vi "BMU诊断标定.vi"(8 "CAN端口":u16(ring), 9 "设备索引号":u16(ring), 10 "CAN卡类型":u32(ring)=21) -> ()   [LabVIEW 2013] (continued)
                n2409 = local write "正级继电器 9"(w2970) -> ()
                n2410 = local write "主从选择"(enum32{"主板", "从板"}."主板" ("主从选择")) -> ()
              }
              frame #1 {
                n2411 = case shown="真" w2980 {
                  selector: w2980 -> [w2995 w3015]
                  tunnel: [w2994 w3014] -> w2979
                  tunnel: [w2982 w3002] -> w2974
                  frame False {
                    w2990 = 256.0 ("y")
                    w2982 = u32 2 ("命令序号")
                    w2994 = u8 192 ("命令")
                    n2412 = local read "动作保持时间"() -> (w2991:dbl)
                    n2413 = Quotient & Remainder(x=w2991, y=w2990) -> (x-y*floor(x/y)=w2983:dbl, floor(x/y)=w2987:dbl)
                    n2414 = Quotient & Remainder(x=w2987, y=w2990) -> (x-y*floor(x/y)=w2984:dbl, floor(x/y)=w2988:dbl)
                    n2415 = Quotient & Remainder(x=w2988, y=w2990) -> (x-y*floor(x/y)=w2985:dbl, floor(x/y)=w2989:dbl)
                    n2416 = local read "设备索引号"() -> (w2999:u16)
                    n2417 = local read "CAN卡类型"() -> (w3000:u32)
                    n2418 = local read "CAN端口"() -> (w2998:u16)
                    n2419 = Boolean To (0,1)(Boolean=w2995) -> (0, 1=w2992:i16)
                    n2420 = Quotient & Remainder(x=w2989, y=w2990) -> (x-y*floor(x/y)=w2986:dbl)  [unwired: 1 out]
                    n2421 = Build Array(i16 1 ("元素"), w2992, w2986, w2985, w2984, w2983, 0.0 ("元素")) -> (w2996:dbl[])
                    n2422 = call "多帧发送机制(EV05).vi"("can卡类型"=w3000, "设备索引号"=w2999, "CAN端口"=w2998, "命令"=w2994, "板号"=u8 0, "命令序号"=w2982, "输入数据"=w2996) -> ()  [unwired: 1 in, 12 out]
                  }
                  frame True {
                    w3010 = 256.0 ("y")
                    w3002 = u32 2 ("命令序号")
                    w3014 = u8 192 ("命令")
                    n2423 = local read "动作保持时间"() -> (w3011:dbl)
                    n2424 = Quotient & Remainder(x=w3011, y=w3010) -> (x-y*floor(x/y)=w3003:dbl, floor(x/y)=w3007:dbl)
                    n2425 = Quotient & Remainder(x=w3007, y=w3010) -> (x-y*floor(x/y)=w3004:dbl, floor(x/y)=w3008:dbl)
                    n2426 = Quotient & Remainder(x=w3008, y=w3010) -> (x-y*floor(x/y)=w3005:dbl, floor(x/y)=w3009:dbl)
                    n2427 = local read "设备索引号"() -> (w3019:u16)
                    n2428 = local read "CAN卡类型"() -> (w3020:u32)
                    n2429 = local read "CAN端口"() -> (w3018:u16)
                    n2430 = Boolean To (0,1)(Boolean=w3015) -> (0, 1=w3012:i16)
                    n2431 = Quotient & Remainder(x=w3009, y=w3010) -> (x-y*floor(x/y)=w3006:dbl)  [unwired: 1 out]
                    n2432 = Build Array(i16 1 ("元素"), w3012, w3006, w3005, w3004, w3003, 0.0 ("元素")) -> (w3016:dbl[])
                    n2433 = call "多帧发送机制(EV05).vi"("can卡类型"=w3020, "设备索引号"=w3019, "CAN端口"=w3018, "命令"=w3014, "板号"=u8 0, "命令序号"=w3002, "输入数据"=w3016) -> ()  [unwired: 1 in, 12 out]
                  }
                }
                n2434 = local write "命令序号"(w2974) -> ()
                n2435 = local write "命令"(w2979) -> ()
                n2436 = local write "控制1"(TRUE ("控制1")) -> ()
                n2437 = local write "写?"(FALSE ("写?")) -> ()
                n2438 = local write "消除"(TRUE ("消除")) -> ()
                n2439 = global write "EV05全局变量1.vi" "流控帧 2"(TRUE ("流控帧 2")) -> ()
                n2440 = global write "EV05全局变量1.vi" "流控帧"(FALSE ("流控帧")) -> ()
              }
              frame #2 {
                n2441 = flat-sequence {
                  tunnel: [w3022] -> w3021
                  tunnel: w3021 -> [w3029]
                  frame #0 {
                    n2442 = while {
                      tunnel: [w3023] -> w3022
                      i -> [w3027]
                      stop <- w3024 stop-if-true
                      n2443 = local read "继电器超时处理"() -> (w3023:bool)
                      n2444 = Greater Or Equal?(x=w3027, y=20) -> (x >= y?=w3025:bool)
                      n2445 = Wait Until Next ms Multiple(millisecond multiple=u32 100 ("毫秒倍数")) -> ()  [unwired: 1 out]
                      n2446 = Or(x=w3023, y=w3025) -> (x .or. y?=w3024:bool)
                    }
                  }
                  frame #1 {
                    n2447 = case shown="假" w3029 {
                      frame False {
                        n2448 = local read "DO1"() -> (w3031:bool)
                        n2449 = Not(x=w3031) -> (.not. x?=w3030:bool)
                        n2450 = local write "DO1"(w3030) -> ()
                        n2451 = One Button Dialog(message="DO控制处理超时" ("消息"), button name ("OK")="是" ("按钮名称（“确定”）")) -> ()  [unwired: 1 out]
                      }
                      frame True {
                      }
                    }
                  }
                }
              }
            }
          }
          event "DO2": Value Change {
            n2452 = event-data() -> ("NewVal"=w3034:bool)  [unwired: 6 out]
            n2453 = stacked-sequence {
              tunnel: w3034 -> [_ w3047 _]
              frame #0 {
                w3037 = FALSE ("清BUFF")
                n2454 = local write "继电器超时处理"(FALSE ("继电器超时处理")) -> ()
                n2455 = local write "主从选择"(enum32{"主板", "从板"}."主板" ("主从选择")) -> ()
                n2456 = local write "清BUFF"(w3037) -> ()
                n2457 = local write "正级继电器 10"(w3037) -> ()
              }
              frame #1 {
                n2458 = case shown="真" w3047 {
                  selector: w3047 -> [w3062 w3082]
                  tunnel: [w3061 w3081] -> w3046
                  tunnel: [w3049 w3069] -> w3041
                  frame False {
                    w3057 = 256.0 ("y")
                    w3049 = u32 2 ("命令序号")
                    w3061 = u8 192 ("命令")
                    n2459 = local read "动作保持时间"() -> (w3058:dbl)
                    n2460 = Quotient & Remainder(x=w3058, y=w3057) -> (x-y*floor(x/y)=w3050:dbl, floor(x/y)=w3054:dbl)
                    n2461 = Quotient & Remainder(x=w3054, y=w3057) -> (x-y*floor(x/y)=w3051:dbl, floor(x/y)=w3055:dbl)
                    n2462 = Quotient & Remainder(x=w3055, y=w3057) -> (x-y*floor(x/y)=w3052:dbl, floor(x/y)=w3056:dbl)
                    n2463 = local read "设备索引号"() -> (w3066:u16)
                    n2464 = local read "CAN卡类型"() -> (w3067:u32)
                    n2465 = local read "CAN端口"() -> (w3065:u16)
                    n2466 = Boolean To (0,1)(Boolean=w3062) -> (0, 1=w3059:i16)
                    n2467 = Quotient & Remainder(x=w3056, y=w3057) -> (x-y*floor(x/y)=w3053:dbl)  [unwired: 1 out]
                    n2468 = Build Array(i16 2 ("元素"), w3059, w3053, w3052, w3051, w3050, 0.0 ("元素")) -> (w3063:dbl[])
                    n2469 = call "多帧发送机制(EV05).vi"("can卡类型"=w3067, "设备索引号"=w3066, "CAN端口"=w3065, "命令"=w3061, "板号"=u8 0, "命令序号"=w3049, "输入数据"=w3063) -> ()  [unwired: 1 in, 12 out]
                  }
                  frame True {
                    w3077 = 256.0 ("y")
                    w3069 = u32 2 ("命令序号")
                    w3081 = u8 192 ("命令")
                    n2470 = local read "动作保持时间"() -> (w3078:dbl)
                    n2471 = Quotient & Remainder(x=w3078, y=w3077) -> (x-y*floor(x/y)=w3070:dbl, floor(x/y)=w3074:dbl)
                    n2472 = Quotient & Remainder(x=w3074, y=w3077) -> (x-y*floor(x/y)=w3071:dbl, floor(x/y)=w3075:dbl)
                    n2473 = Quotient & Remainder(x=w3075, y=w3077) -> (x-y*floor(x/y)=w3072:dbl, floor(x/y)=w3076:dbl)
                    n2474 = local read "设备索引号"() -> (w3086:u16)
                    n2475 = local read "CAN卡类型"() -> (w3087:u32)
                    n2476 = local read "CAN端口"() -> (w3085:u16)
                    n2477 = Boolean To (0,1)(Boolean=w3082) -> (0, 1=w3079:i16)
                    n2478 = Quotient & Remainder(x=w3076, y=w3077) -> (x-y*floor(x/y)=w3073:dbl)  [unwired: 1 out]
                    n2479 = Build Array(i16 2 ("元素"), w3079, w3073, w3072, w3071, w3070, 0.0 ("元素")) -> (w3083:dbl[])
                    n2480 = call "多帧发送机制(EV05).vi"("can卡类型"=w3087, "设备索引号"=w3086, "CAN端口"=w3085, "命令"=w3081, "板号"=u8 0, "命令序号"=w3069, "输入数据"=w3083) -> ()  [unwired: 1 in, 12 out]
                  }
                }
                n2481 = local write "命令序号"(w3041) -> ()
                n2482 = local write "命令"(w3046) -> ()
                n2483 = local write "控制1"(TRUE ("控制1")) -> ()
                n2484 = local write "写?"(FALSE ("写?")) -> ()
                n2485 = local write "消除"(TRUE ("消除")) -> ()
                n2486 = global write "EV05全局变量1.vi" "流控帧 2"(TRUE ("流控帧 2")) -> ()
                n2487 = global write "EV05全局变量1.vi" "流控帧"(FALSE ("流控帧")) -> ()
              }
              frame #2 {
                n2488 = flat-sequence {
                  tunnel: [w3089] -> w3088
                  tunnel: w3088 -> [w3096]
                  frame #0 {
                    n2489 = while {
                      tunnel: [w3090] -> w3089
                      i -> [w3094]
                      stop <- w3091 stop-if-true
                      n2490 = local read "继电器超时处理"() -> (w3090:bool)
                      n2491 = Greater Or Equal?(x=w3094, y=20) -> (x >= y?=w3092:bool)
                      n2492 = Wait Until Next ms Multiple(millisecond multiple=u32 100 ("毫秒倍数")) -> ()  [unwired: 1 out]
                      n2493 = Or(x=w3090, y=w3092) -> (x .or. y?=w3091:bool)
                    }
                  }
                  frame #1 {
                    n2494 = case shown="假" w3096 {
                      frame False {
                        n2495 = local read "DO2"() -> (w3098:bool)
                        n2496 = Not(x=w3098) -> (.not. x?=w3097:bool)
                        n2497 = local write "DO2"(w3097) -> ()
                        n2498 = One Button Dialog(message="DO控制处理超时" ("消息"), button name ("OK")="是" ("按钮名称（“确定”）")) -> ()  [unwired: 1 out]
                      }
                      frame True {
                      }
                    }
                  }
                }
              }
            }
          }
          event "DO1 2": Value Change {
            n2499 = event-data() -> ("NewVal"=w3101:bool)  [unwired: 6 out]
            n2500 = stacked-sequence {
              tunnel: w3101 -> [_ w3115 _]
              frame #0 {
                w3104 = FALSE ("继电器超时处理")
                n2501 = local write "继电器超时处理"(w3104) -> ()
                n2502 = local write "正级继电器 11"(w3104) -> ()
                n2503 = local write "主从选择"(enum32{"主板", "从板"}."从板" ("主从选择")) -> ()
              }
              frame #1 {
                n2504 = case shown="假" w3115 {
                  selector: w3115 -> [w3130 w3150]
                  tunnel: [w3129 w3149] -> w3114
                  tunnel: [w3128 w3148] -> w3108
                  tunnel: [w3117 w3137] -> w3109
                  frame True {
                    w3125 = 256.0 ("y")
                    w3117 = u32 2 ("命令序号")
                    w3129 = u8 192 ("命令")
                    n2505 = local read "动作保持时间"() -> (w3126:dbl)
                    n2506 = Quotient & Remainder(x=w3126, y=w3125) -> (x-y*floor(x/y)=w3118:dbl, floor(x/y)=w3122:dbl)
                    n2507 = Quotient & Remainder(x=w3122, y=w3125) -> (x-y*floor(x/y)=w3119:dbl, floor(x/y)=w3123:dbl)
                    n2508 = Quotient & Remainder(x=w3123, y=w3125) -> (x-y*floor(x/y)=w3120:dbl, floor(x/y)=w3124:dbl)
                    n2509 = Quotient & Remainder(x=w3124, y=w3125) -> (x-y*floor(x/y)=w3121:dbl)  [unwired: 1 out]
                    n2510 = Boolean To (0,1)(Boolean=w3130) -> (0, 1=w3127:i16)
                    n2511 = local read "设备索引号"() -> (w3134:u16)
                    n2512 = local read "CAN卡类型"() -> (w3135:u32)
                    n2513 = local read "从板板号"() -> (w3128:u8)
                    n2514 = local read "CAN端口"() -> (w3133:u16)
                    n2515 = Build Array(i16 3 ("元素"), w3127, w3121, w3120, w3119, w3118, 0.0 ("元素")) -> (w3132:dbl[])
                    n2516 = call "多帧发送机制(EV05).vi"("can卡类型"=w3135, "设备索引号"=w3134, "CAN端口"=w3133, "命令"=w3129, "板号"=w3128, "命令序号"=w3117, "输入数据"=w3132) -> ()  [unwired: 1 in, 12 out]
                  }
                  frame False {
                    w3145 = 256.0 ("y")
                    w3137 = u32 2 ("命令序号")
                    w3149 = u8 192 ("命令")
                    n2517 = local read "动作保持时间"() -> (w3146:dbl)
                    n2518 = Quotient & Remainder(x=w3146, y=w3145) -> (x-y*floor(x/y)=w3138:dbl, floor(x/y)=w3142:dbl)
                    n2519 = Quotient & Remainder(x=w3142, y=w3145) -> (x-y*floor(x/y)=w3139:dbl, floor(x/y)=w3143:dbl)
                    n2520 = Quotient & Remainder(x=w3143, y=w3145) -> (x-y*floor(x/y)=w3140:dbl, floor(x/y)=w3144:dbl)
                    n2521 = Quotient & Remainder(x=w3144, y=w3145) -> (x-y*floor(x/y)=w3141:dbl)  [unwired: 1 out]
                    n2522 = Boolean To (0,1)(Boolean=w3150) -> (0, 1=w3147:i16)
                    n2523 = local read "设备索引号"() -> (w3154:u16)
                    n2524 = local read "CAN卡类型"() -> (w3155:u32)
                    n2525 = local read "从板板号"() -> (w3148:u8)
                    n2526 = local read "CAN端口"() -> (w3153:u16)
                    n2527 = Build Array(i16 1 ("元素"), w3147, w3141, w3140, w3139, w3138, 0.0 ("元素")) -> (w3152:dbl[])
                    n2528 = call "多帧发送机制(EV05).vi"("can卡类型"=w3155, "设备索引号"=w3154, "CAN端口"=w3153, "命令"=w3149, "板号"=w3148, "命令序号"=w3137, "输入数据"=w3152) -> ()  [unwired: 1 in, 12 out]
                  }
                }
                n2529 = local write "从板板号"(w3108) -> ()
                n2530 = local write "命令序号"(w3109) -> ()
                n2531 = local write "命令"(w3114) -> ()
                n2532 = local write "清BUFF"(FALSE ("清BUFF")) -> ()
                n2533 = local write "写?"(FALSE ("写?")) -> ()
                n2534 = local write "控制1"(TRUE ("控制1")) -> ()
                n2535 = global write "EV05全局变量1.vi" "流控帧"(FALSE ("流控帧")) -> ()
                n2536 = global write "EV05全局变量1.vi" "流控帧 2"(TRUE ("流控帧 2")) -> ()
                n2537 = local write "消除"(TRUE ("消除")) -> ()
              }
              frame #2 {
                n2538 = flat-sequence {
                  tunnel: [w3157] -> w3156
                  tunnel: w3156 -> [w3164]
                  frame #0 {
                    n2539 = while {
                      tunnel: [w3158] -> w3157
                      i -> [w3162]
                      stop <- w3159 stop-if-true
                      n2540 = local read "继电器超时处理"() -> (w3158:bool)
                      n2541 = Greater Or Equal?(x=w3162, y=20) -> (x >= y?=w3160:bool)
                      n2542 = Wait Until Next ms Multiple(millisecond multiple=u32 100 ("毫秒倍数")) -> ()  [unwired: 1 out]
                      n2543 = Or(x=w3158, y=w3160) -> (x .or. y?=w3159:bool)
                    }
                  }
                  frame #1 {
                    n2544 = case shown="假" w3164 {
                      frame False {
                        n2545 = local read "DO1 2"() -> (w3166:bool)
                        n2546 = Not(x=w3166) -> (.not. x?=w3165:bool)
                        n2547 = local write "DO1 2"(w3165) -> ()
                        n2548 = One Button Dialog(message="DO控制处理超时" ("消息"), button name ("OK")="是" ("按钮名称（“确定”）")) -> ()  [unwired: 1 out]
                      }
                      frame True {
                      }
                    }
                  }
                }
              }
            }
          }
          event "读取转换为写入": Value Change {
            n2549 = event-data() -> ("NewVal"=w3169:bool)  [unwired: 6 out]
            n2550 = case shown="真" w3169 {
              tunnel: w3173 -> [w3175 w3180]
              tunnel: [w3175 w3179] -> w3172
              tunnel: w3171 -> [w3174 w3178]
              tunnel: [w3174 w3177] -> w3170
              frame False {
              }
              frame True {
                n2551 = Enqueue Element(queue=w3180, element="读取转换为写入", error in (no error)=w3178) -> (queue out=w3179:refnum<queue>, error out=w3177:errorcluster)  [unwired: 2 out]
              }
            }
          }
          event "读取故障详细状态": Value Change {
            n2552 = event-data() -> ("NewVal"=w3185:bool)  [unwired: 5 out]
            n2553 = case shown="真" w3185 {
              tunnel: w3184 -> [w3187 w3200]
              tunnel: w3183 -> [w3186 w3199]
              tunnel: [w3187 w3198] -> w3182
              tunnel: [w3186 w3197] -> w3181
              frame False {
              }
              frame True {
                n2554 = disable-structure shown="启用" {
                  disable-tunnel: [w3209 TRUE ("发送成功")] -> w3196
                  frame Disabled {
                    n2555 = local read "主从选择"() -> (w3201:enum32{"主板", "从板"})
                    n2556 = case shown="\"主板\", 默认" w3201 {
                      tunnel: [0.0 ("FUNC") w3211] -> w3206
                      frame "主板", Default {
                      }
                      frame "从板" {
                        n2557 = local read "从板号"() -> (w3211:u8)
                      }
                    }
                    n2558 = local read "设备索引号"() -> (w3203:u16)
                    n2559 = local read "CAN卡类型"() -> (w3204:u32)
                    n2560 = local read "CAN端口"() -> (w3202:u16)
                    n2561 = call "标定授权发送.vi"("CAN卡类型"=w3204, "解锁类型"=enum16{"读取", "写", "下载"}."写", "设备索引号"=w3203, "CAN端口"=w3202, "是否连接"=TRUE, "板选择"=0, "FUNC"=w3206) -> ("发送成功"=w3209:bool)  [unwired: 8 out]
                  }
                  frame Enabled {
                  }
                }
                n2562 = case shown="真" w3196 {
                  tunnel: w3200 -> [w3214 w3219]
                  tunnel: w3199 -> [w3213 w3218]
                  tunnel: [w3214 w3216] -> w3198
                  tunnel: [w3213 w3215] -> w3197
                  frame False {
                  }
                  frame True {
                    n2563 = Enqueue Element(queue=w3219, element="读取故障状态" ("元素"), error in (no error)=w3218) -> (queue out=w3216:refnum<queue>, error out=w3215:errorcluster)  [unwired: 2 out]
                  }
                }
                n2564 = local write "电池故障"(string[][] []) -> ()
                n2565 = global write "EV05全局变量1.vi" "流控帧 2"(TRUE ("流控帧")) -> ()
                n2566 = local write "写?"(FALSE ("写?")) -> ()
                n2567 = local write "控制1"(TRUE ("控制1")) -> ()
                n2568 = local write "消除"(TRUE ("消除")) -> ()
                n2569 = local write "清BUFF"(FALSE ("清BUFF")) -> ()
                n2570 = global write "EV05全局变量1.vi" "流控帧"(FALSE ("流控帧")) -> ()
                n2571 = call <vilib>:"Set Busy.vi"("disable click? (T)"=FALSE) -> ()  [unwired: 3 in, 8 out]
              }
            }
          }
          event "项目软本读取": Value Change {
            n2572 = event-data() -> ("NewVal"=w3224:bool)  [unwired: 5 out]
            n2573 = case shown="真" w3224 {
              tunnel: w3223 -> [w3226 w3233]
              tunnel: w3222 -> [w3225 w3232]
              tunnel: [w3226 w3231] -> w3221
              tunnel: [w3225 w3230] -> w3220
              frame False {
              }
              frame True {
                n2574 = global read "EV05全局变量1.vi" "授权功能"() -> (w3228:bool)
                n2575 = case shown="假" w3228 {
                  tunnel: [TRUE ("发送成功") w3252] -> w3229
                  frame False {
                  }
                  frame True {
                    n2576 = local read "设备索引号"() -> (w3247:u16)
                    n2577 = local read "CAN卡类型"() -> (w3248:u32)
                    n2578 = local read "CAN端口"() -> (w3246:u16)
                    n2579 = call "标定授权发送.vi"("CAN卡类型"=w3248, "解锁类型"=enum16{"读取", "写", "下载"}."读取", "设备索引号"=w3247, "CAN端口"=w3246, "是否连接"=TRUE, "板选择"=0, "FUNC"=u32 0) -> ("发送成功"=w3252:bool)  [unwired: 8 out]
                  }
                }
                n2580 = stacked-sequence {
                  tunnel: [w3236] -> w3227
                  frame #0 {
                    w3236 = FALSE ("disable click? (T)")
                    w3239 = FALSE ("写?")
                    n2581 = local write "写?"(w3239) -> ()
                    n2582 = global write "EV05全局变量1.vi" "写入超时"(w3239) -> ()
                    n2583 = local write "项目软件版本号"(" " ("项目软件版本号")) -> ()
                    n2584 = global write "EV05全局变量1.vi" "流控帧"(FALSE ("流控帧")) -> ()
                    n2585 = local write "主从选择"(enum32{"主板", "从板"}."主板" ("主从选择")) -> ()
                    n2586 = call <vilib>:"Set Busy.vi"("disable click? (T)"=w3236) -> ()  [unwired: 3 in, 8 out]
                    n2587 = local write "清BUFF"(FALSE ("清BUFF")) -> ()
                    n2588 = property on="保存版本信息" class="Bool (严格)"("Visible"=TRUE ("可见")) -> ()  [unwired: 2 in, 2 out]
                    n2589 = global write "EV05全局变量1.vi" "流控帧 2"(TRUE ("流控帧 2")) -> ()
                    n2590 = local write "控制1"(TRUE ("控制1")) -> ()
                    n2591 = local write "消除"(TRUE ("消除")) -> ()
                  }
                }
                n2592 = case shown="真" w3229 {
                  tunnel: w3233 -> [w3254 w3259]
                  tunnel: w3232 -> [w3253 w3258]
                  tunnel: [w3254 w3256] -> w3231
                  tunnel: [w3253 w3255] -> w3230
                  tunnel: w3227 -> [_ _]
                  frame False {
                  }
                  frame True {
                    n2593 = Enqueue Element(queue=w3259, element="项目软件版本读取" ("元素"), error in (no error)=w3258) -> (queue out=w3256:refnum<queue>, error out=w3255:errorcluster)  [unwired: 2 out]
                  }
                }
              }
            }
          }
          event "读硬件版本号": Value Change {
            n2594 = event-data() -> ("NewVal"=w3264:bool)  [unwired: 5 out]
            n2595 = case shown="真" w3264 {
              tunnel: w3263 -> [w3266 w3273]
              tunnel: w3262 -> [w3265 w3272]
              tunnel: [w3266 w3271] -> w3261
              tunnel: [w3265 w3270] -> w3260
              frame False {
              }
              frame True {
                n2596 = global read "EV05全局变量1.vi" "授权功能"() -> (w3268:bool)
                n2597 = case shown="假" w3268 {
                  tunnel: [TRUE ("发送成功") w3292] -> w3269
                  frame False {
                  }
                  frame True {
                    n2598 = local read "设备索引号"() -> (w3287:u16)
                    n2599 = local read "CAN卡类型"() -> (w3288:u32)
                    n2600 = local read "CAN端口"() -> (w3286:u16)
                    n2601 = call "标定授权发送.vi"("CAN卡类型"=w3288, "解锁类型"=enum16{"读取", "写", "下载"}."读取", "设备索引号"=w3287, "CAN端口"=w3286, "是否连接"=TRUE, "板选择"=0, "FUNC"=u32 0) -> ("发送成功"=w3292:bool)  [unwired: 8 out]
                  }
                }
                n2602 = stacked-sequence {
                  tunnel: [w3276] -> w3267
                  frame #0 {
                    w3276 = TRUE ("控制1")
                    w3280 = FALSE ("写?")
                    n2603 = local write "写?"(w3280) -> ()
                    n2604 = global write "EV05全局变量1.vi" "写入超时"(w3280) -> ()
                    n2605 = call <vilib>:"Set Busy.vi"("disable click? (T)"=FALSE) -> ()  [unwired: 3 in, 8 out]
                    n2606 = local write "硬件版本号"("" ("硬件版本号")) -> ()
                    n2607 = property on="保存版本信息" class="Bool (严格)"("Visible"=TRUE ("可见")) -> ()  [unwired: 2 in, 2 out]
                    n2608 = local write "主从选择"(enum32{"主板", "从板"}."主板" ("主从选择")) -> ()
                    n2609 = local write "控制1"(w3276) -> ()
                    n2610 = local write "清BUFF"(FALSE ("清BUFF")) -> ()
                    n2611 = global write "EV05全局变量1.vi" "流控帧 2"(TRUE ("流控帧 2")) -> ()
                    n2612 = local write "消除"(TRUE ("消除")) -> ()
                    n2613 = global write "EV05全局变量1.vi" "流控帧"(FALSE ("流控帧")) -> ()
                  }
                }
                n2614 = case shown="真" w3269 {
                  tunnel: w3273 -> [w3294 w3299]
                  tunnel: w3272 -> [w3293 w3298]
                  tunnel: [w3294 w3296] -> w3271
                  tunnel: [w3293 w3295] -> w3270
                  tunnel: w3267 -> [_ _]
                  frame False {
                  }
                  frame True {
                    n2615 = Enqueue Element(queue=w3299, element="硬件版本读取" ("元素"), error in (no error)=w3298) -> (queue out=w3296:refnum<queue>, error out=w3295:errorcluster)  [unwired: 2 out]
                  }
                }
              }
            }
          }
          event "平台软件版本读取": Value Change {
            n2616 = event-data() -> ("NewVal"=w3304:bool)  [unwired: 5 out]
            n2617 = case shown="真" w3304 {
              tunnel: w3303 -> [w3306 w3313]
              tunnel: w3302 -> [w3305 w3312]
              tunnel: [w3306 w3311] -> w3301
              tunnel: [w3305 w3310] -> w3300
              frame False {
              }
              frame True {
                n2618 = global read "EV05全局变量1.vi" "授权功能"() -> (w3308:bool)
                n2619 = case shown="假" w3308 {
                  tunnel: [TRUE ("发送成功") w3332] -> w3309
                  frame False {
                  }
                  frame True {
                    n2620 = local read "设备索引号"() -> (w3327:u16)
                    n2621 = local read "CAN卡类型"() -> (w3328:u32)
                    n2622 = local read "CAN端口"() -> (w3326:u16)
                    n2623 = call "标定授权发送.vi"("CAN卡类型"=w3328, "解锁类型"=enum16{"读取", "写", "下载"}."读取", "设备索引号"=w3327, "CAN端口"=w3326, "是否连接"=TRUE, "板选择"=0, "FUNC"=u32 0) -> ("发送成功"=w3332:bool)  [unwired: 8 out]
                  }
                }
                n2624 = stacked-sequence {
                  tunnel: [w3316] -> w3307
                  frame #0 {
                    w3316 = TRUE ("控制1")
                    w3320 = FALSE ("写?")
                    n2625 = call <vilib>:"Set Busy.vi"("disable click? (T)"=FALSE) -> ()  [unwired: 3 in, 8 out]
                    n2626 = local write "写?"(w3320) -> ()
                    n2627 = global write "EV05全局变量1.vi" "写入超时"(w3320) -> ()
                    n2628 = local write "平台软件版本号"(" " ("平台软件版本号")) -> ()
                    n2629 = local write "控制1"(w3316) -> ()
                    n2630 = local write "消除"(TRUE ("消除")) -> ()
                    n2631 = property on="保存版本信息" class="Bool (严格)"("Visible"=TRUE ("可见")) -> ()  [unwired: 2 in, 2 out]
                    n2632 = global write "EV05全局变量1.vi" "流控帧 2"(TRUE ("流控帧 2")) -> ()
                    n2633 = local write "主从选择"(enum32{"主板", "从板"}."主板" ("主从选择")) -> ()
                    n2634 = local write "清BUFF"(FALSE ("清BUFF")) -> ()
                    n2635 = global write "EV05全局变量1.vi" "流控帧"(FALSE ("流控帧")) -> ()
                  }
                }
                n2636 = case shown="真" w3309 {
                  tunnel: w3313 -> [w3334 w3339]
                  tunnel: w3312 -> [w3333 w3338]
                  tunnel: [w3334 w3336] -> w3311
                  tunnel: [w3333 w3335] -> w3310
                  tunnel: w3307 -> [_ _]
                  frame False {
                  }
                  frame True {
                    n2637 = Enqueue Element(queue=w3339, element="平台软件版本读取" ("元素"), error in (no error)=w3338) -> (queue out=w3336:refnum<queue>, error out=w3335:errorcluster)  [unwired: 2 out]
                  }
                }
              }
            }
          }
          event "模块版本读取": Value Change {
            n2638 = event-data() -> ("NewVal"=w3344:bool)  [unwired: 5 out]
            n2639 = case shown="真" w3344 {
              tunnel: w3343 -> [w3346 w3353]
              tunnel: w3342 -> [w3345 w3352]
              tunnel: [w3346 w3351] -> w3341
              tunnel: [w3345 w3350] -> w3340
              frame False {
              }
              frame True {
                n2640 = global read "EV05全局变量1.vi" "授权功能"() -> (w3348:bool)
                n2641 = case shown="假" w3348 {
                  tunnel: [TRUE ("发送成功") w3371] -> w3349
                  frame False {
                  }
                  frame True {
                    n2642 = local read "设备索引号"() -> (w3366:u16)
                    n2643 = local read "CAN卡类型"() -> (w3367:u32)
                    n2644 = local read "CAN端口"() -> (w3365:u16)
                    n2645 = call "标定授权发送.vi"("CAN卡类型"=w3367, "解锁类型"=enum16{"读取", "写", "下载"}."读取", "设备索引号"=w3366, "CAN端口"=w3365, "是否连接"=TRUE, "板选择"=0, "FUNC"=u32 0) -> ("发送成功"=w3371:bool)  [unwired: 8 out]
                  }
                }
                n2646 = stacked-sequence {
                  tunnel: [w3356] -> w3347
                  frame #0 {
                    w3356 = TRUE ("控制1")
                    w3359 = FALSE ("写?")
                    n2647 = call <vilib>:"Set Busy.vi"("disable click? (T)"=FALSE) -> ()  [unwired: 3 in, 8 out]
                    n2648 = local write "写?"(w3359) -> ()
                    n2649 = global write "EV05全局变量1.vi" "写入超时"(w3359) -> ()
                    n2650 = local write "主从选择"(enum32{"主板", "从板"}."主板" ("主从选择")) -> ()
                    n2651 = local write "清BUFF"(FALSE ("清BUFF")) -> ()
                    n2652 = property on="保存版本信息" class="Bool (严格)"("Visible"=TRUE ("可见")) -> ()  [unwired: 2 in, 2 out]
                    n2653 = global write "EV05全局变量1.vi" "流控帧 2"(TRUE ("流控帧 2")) -> ()
                    n2654 = local write "控制1"(w3356) -> ()
                    n2655 = local write "消除"(TRUE ("消除")) -> ()
                    n2656 = global write "EV05全局变量1.vi" "流控帧"(FALSE ("流控帧")) -> ()
                  }
                }
                n2657 = case shown="真" w3349 {
                  tunnel: w3353 -> [w3373 w3378]
                  tunnel: w3352 -> [w3372 w3377]
                  tunnel: [w3373 w3375] -> w3351
                  tunnel: [w3372 w3374] -> w3350
                  tunnel: w3347 -> [_ _]
                  frame False {
                  }
                  frame True {
                    n2658 = Enqueue Element(queue=w3378, element="模块软件版本读取" ("元素"), error in (no error)=w3377) -> (queue out=w3375:refnum<queue>, error out=w3374:errorcluster)  [unwired: 2 out]
                  }
                }
              }
            }
          }
          event "保存版本信息": Value Change {
            n2659 = event-data() -> ("NewVal"=w3379:bool)  [unwired: 6 out]
            n2660 = case shown="真" w3379 {
              frame False {
              }
              frame True {
                n2661 = stacked-sequence {
                  seq-local: [w3383 _] -> [_ w3385]
                  seq-local: [w3382 _] -> [_ w3384]
                  frame #0 {
                    n2662 = call "请输入从板个数"() -> ("从板个数"=w3383:dbl, "确定"=w3382:bool)  [unwired: 17 in, 1 out]
                  }
                  frame #1 {
                    n2663 = case shown="真" w3384 {
                      tunnel: w3385 -> [_ w3388]
                      frame False {
                      }
                      frame True {
                        n2664 = call <vilib>:"Application Directory.vi"() -> ("Application Directory"=w3400:path)
                        n2665 = Build Path(base path=w3400, name or relative path="SaveData" ("名称或相对路径")) -> (appended path=w3398:path)
                        n2666 = local read "模块版本名称"() -> (w3393:string[][])
                        n2667 = local read "项目软件版本"() -> (w3390:string[])
                        n2668 = local read "模块版本值"() -> (w3392:string[][])
                        n2669 = local read "平台软件版本"() -> (w3389:string[])
                        n2670 = local read "模块个数"() -> (w3386:u8[])
                        n2671 = local read "硬件版本"() -> (w3391:string[])
                        n2672 = call "文件对话框3"("start path"=w3398, "prompt"="选择要保存数据的位置", "default name"="BMS版本信息.txt") -> ("selected path"=w3394:path, "cancelled"=w3395:bool)  [unwired: 9 in, 2 out]
                        n2673 = Increment(x=w3388) -> (x+1=w3387:dbl)
                        n2674 = for {
                          N: w3387 -> [_]
                          tunnel: w3395 -> [w3416]
                          tunnel: w3394 -> [w3415]
                          tunnel: w3393 -> [w3405] mode=indexing
                          tunnel: w3392 -> [w3403] mode=indexing
                          tunnel: w3391 -> [w3410] mode=indexing
                          tunnel: w3390 -> [w3409] mode=indexing
                          tunnel: w3389 -> [w3408] mode=indexing
                          tunnel: w3386 -> [w3401] mode=indexing
                          i -> [w3407]
                          w3413 = ""
                          w3420 = 0 ("索引")
                          n2675 = case shown="0, 默认" w3407 {
                            selector: w3407 -> [_ w3434]
                            tunnel: ["主板版本信息" w3435] -> w3425
                            tunnel: [FALSE TRUE] -> w3411
                            frame 0, Default {
                            }
                            frame 1.. {
                              n2676 = Number To Decimal String(number=w3434) -> (decimal integer string=w3433:string)  [unwired: 1 in]
                              n2677 = Concatenate Strings("从板", w3433, "版本信息") -> (w3435:string)
                            }
                          }
                          n2678 = Increment(x=w3401) -> (x+1=w3402:u8)
                          n2679 = Array Subset(array=w3405, length=w3402) -> (w3406:string[])  [unwired: 1 in]
                          n2680 = Array Subset(array=w3403, length=w3402) -> (w3404:string[])  [unwired: 1 in]
                          n2681 = Build Array(w3413, w3408, w3409, w3410, w3413) -> (w3419:string[])
                          n2682 = Build Array(w3425, "平台软件版本号", "项目软件版本号", "硬件版本号", "模块版本号") -> (w3421:string[])
                          n2683 = Insert Into Array(array=w3406, index=w3420, new element=w3421) -> (w3418:string[])
                          n2684 = Insert Into Array(array=w3404, index=w3420, new element=w3419) -> (w3417:string[])
                          n2685 = Build Array(w3418, w3417) -> (w3414:string[][])
                          n2686 = case shown="假" w3416 {
                            tunnel: w3415 -> [w3429 _]
                            tunnel: w3414 -> [w3428 _]
                            tunnel: w3411 -> [w3426 _]
                            frame False {
                              n2687 = call-poly <vilib>:"Write To Spreadsheet File.vi"("transpose? (no:F)"=TRUE, "append to file? (new file:F)"=w3426, "2D data"=w3428, "file path (dialog if empty)"=w3429) -> ()  [unwired: 4 in, 1 out]
                            }
                            frame True {
                            }
                          }
                        }
                      }
                    }
                  }
                }
              }
            }
          }
          event "单个写入": Value Change {
            n2688 = event-data() -> ("NewVal"=w3442:bool)  [unwired: 5 out]
            n2689 = case shown="真" w3442 {
              tunnel: w3441 -> [w3444 w3451]
              tunnel: w3440 -> [w3443 w3450]
              tunnel: [w3444 w3449] -> w3439
              tunnel: [w3443 w3448] -> w3438
              frame False {
              }
              frame True {
                w3446 = FALSE ("流控帧")
                w3445 = TRUE ("流控帧 2")
                n2690 = disable-structure shown="启用" {
                  disable-tunnel: [w3460 TRUE ("发送成功")] -> w3447
                  frame Disabled {
                    n2691 = local read "主从选择"() -> (w3452:enum32{"主板", "从板"})
                    n2692 = case shown="\"主板\", 默认" w3452 {
                      tunnel: [0.0 ("FUNC") w3462] -> w3457
                      frame "主板", Default {
                      }
                      frame "从板" {
                        n2693 = local read "从板号"() -> (w3462:u8)
                      }
                    }
                    n2694 = local read "设备索引号"() -> (w3454:u16)
                    n2695 = local read "CAN卡类型"() -> (w3455:u32)
                    n2696 = local read "CAN端口"() -> (w3453:u16)
                    n2697 = call "标定授权发送.vi"("CAN卡类型"=w3455, "解锁类型"=enum16{"读取", "写", "下载"}."写", "设备索引号"=w3454, "CAN端口"=w3453, "是否连接"=TRUE, "板选择"=0, "FUNC"=w3457) -> ("发送成功"=w3460:bool)  [unwired: 8 out]
                  }
                  frame Enabled {
                  }
                }
                n2698 = case shown="真" w3447 {
                  tunnel: w3451 -> [w3465 w3469]
                  tunnel: w3450 -> [w3464 w3468]
                  tunnel: [w3465 w3471] -> w3449
                  tunnel: [w3464 w3470] -> w3448
                  frame False {
                  }
                  frame True {
                    n2699 = Flush Queue(queue=w3469, error in (no error)=w3468) -> (queue out=w3467:refnum<queue>, error out=w3466:errorcluster)  [unwired: 1 out]
                    n2700 = Enqueue Element(queue=w3467, element="单个写入" ("元素"), error in (no error)=w3466) -> (queue out=w3471:refnum<queue>, error out=w3470:errorcluster)  [unwired: 2 out]
                  }
                }
                n2701 = global write "EV05全局变量1.vi" "读取超时"(w3446) -> ()
                n2702 = global write "EV05全局变量1.vi" "流控帧"(w3446) -> ()
                n2703 = local write "消除"(w3445) -> ()
                n2704 = local write "控制1"(w3445) -> ()
                n2705 = global write "EV05全局变量1.vi" "流控帧 2"(w3445) -> ()
                n2706 = local write "写?"(w3445) -> ()
              }
            }
          }
          event "全部写入": Value Change {
            n2707 = event-data() -> ("NewVal"=w3477:bool)  [unwired: 5 out]
            n2708 = case shown="真" w3477 {
              tunnel: w3476 -> [w3479 w3487]
              tunnel: w3475 -> [w3478 w3486]
              tunnel: [w3479 w3485] -> w3474
              tunnel: [w3478 w3484] -> w3473
              frame False {
              }
              frame True {
                w3481 = FALSE ("流控帧")
                w3480 = TRUE ("流控帧 2")
                n2709 = global read "EV05全局变量1.vi" "授权功能"() -> (w3482:bool)
                n2710 = case shown="真" w3482 {
                  tunnel: [TRUE ("发送成功") w3497] -> w3483
                  frame False {
                  }
                  frame True {
                    n2711 = local read "主从选择"() -> (w3489:enum32{"主板", "从板"})
                    n2712 = case shown="\"从板\"" w3489 {
                      tunnel: [0.0 ("FUNC") w3499] -> w3490
                      frame "主板", Default {
                      }
                      frame "从板" {
                        n2713 = local read "从板号"() -> (w3499:u8)
                      }
                    }
                    n2714 = local read "设备索引号"() -> (w3492:u16)
                    n2715 = local read "CAN卡类型"() -> (w3493:u32)
                    n2716 = local read "CAN端口"() -> (w3491:u16)
                    n2717 = call "标定授权发送.vi"("CAN卡类型"=w3493, "解锁类型"=enum16{"读取", "写", "下载"}."写", "设备索引号"=w3492, "CAN端口"=w3491, "是否连接"=TRUE, "板选择"=0, "FUNC"=w3490) -> ("发送成功"=w3497:bool)  [unwired: 8 out]
                  }
                }
                n2718 = case shown="真" w3483 {
                  tunnel: w3487 -> [w3501 w3505]
                  tunnel: w3486 -> [w3500 w3504]
                  tunnel: [w3501 w3507] -> w3485
                  tunnel: [w3500 w3506] -> w3484
                  frame False {
                  }
                  frame True {
                    n2719 = Flush Queue(queue=w3505, error in (no error)=w3504) -> (queue out=w3503:refnum<queue>, error out=w3502:errorcluster)  [unwired: 1 out]
                    n2720 = Enqueue Element(queue=w3503, element="全部写入" ("元素"), error in (no error)=w3502) -> (queue out=w3507:refnum<queue>, error out=w3506:errorcluster)  [unwired: 1 in, 1 out]
                  }
                }
                n2721 = global write "EV05全局变量1.vi" "读取超时"(w3481) -> ()
                n2722 = global write "EV05全局变量1.vi" "流控帧"(w3481) -> ()
                n2723 = local write "消除"(w3480) -> ()
                n2724 = local write "控制1"(w3480) -> ()
                n2725 = global write "EV05全局变量1.vi" "流控帧 2"(w3480) -> ()
                n2726 = local write "写?"(w3480) -> ()
              }
            }
          }
          event "单个读取": Value Change {
            n2727 = event-data() -> ("NewVal"=w3513:bool)  [unwired: 5 out]
            n2728 = case shown="真" w3513 {
              tunnel: w3512 -> [w3515 w3523]
              tunnel: w3511 -> [w3514 w3522]
              tunnel: [w3515 w3521] -> w3510
              tunnel: [w3514 w3520] -> w3509
              frame False {
              }
              frame True {
                w3516 = FALSE ("流控帧")
                w3517 = TRUE ("流控帧 2")
                n2729 = global read "EV05全局变量1.vi" "授权功能"() -> (w3518:bool)
                n2730 = case shown="假" w3518 {
                  tunnel: [TRUE ("发送成功") w3532] -> w3519
                  frame False {
                  }
                  frame True {
                    n2731 = local read "设备索引号"() -> (w3526:u16)
                    n2732 = local read "CAN卡类型"() -> (w3527:u32)
                    n2733 = local read "CAN端口"() -> (w3525:u16)
                    n2734 = call "标定授权发送.vi"("CAN卡类型"=w3527, "解锁类型"=enum16{"读取", "写", "下载"}."读取", "设备索引号"=w3526, "CAN端口"=w3525, "是否连接"=TRUE, "板选择"=0, "FUNC"=u32 1) -> ("发送成功"=w3532:bool)  [unwired: 8 out]
                  }
                }
                n2735 = case shown="真" w3519 {
                  tunnel: w3523 -> [w3534 w3538]
                  tunnel: w3522 -> [w3533 w3536]
                  tunnel: [w3534 w3540] -> w3521
                  tunnel: [w3533 w3539] -> w3520
                  frame False {
                  }
                  frame True {
                    n2736 = Flush Queue(queue=w3538, error in (no error)=w3536) -> (queue out=w3537:refnum<queue>, error out=w3535:errorcluster)  [unwired: 1 out]
                    n2737 = Enqueue Element(queue=w3537, element="单个读取" ("元素"), error in (no error)=w3535) -> (queue out=w3540:refnum<queue>, error out=w3539:errorcluster)  [unwired: 2 out]
                  }
                }
                n2738 = global write "EV05全局变量1.vi" "写入超时"(w3516) -> ()
                n2739 = global write "EV05全局变量1.vi" "流控帧"(w3516) -> ()
                n2740 = local write "写?"(w3516) -> ()
                n2741 = local write "消除"(w3517) -> ()
                n2742 = local write "控制1"(w3517) -> ()
                n2743 = global write "EV05全局变量1.vi" "流控帧 2"(w3517) -> ()
              }
            }
          }
          event "全部读取": Value Change {
            n2744 = event-data() -> ("NewVal"=w3546:bool)  [unwired: 5 out]
            n2745 = case shown="真" w3546 {
              tunnel: w3545 -> [w3548 w3552]
              tunnel: w3544 -> [w3547 w3551]
              tunnel: [w3548 w3550] -> w3543
              tunnel: [w3547 w3549] -> w3542
              frame False {
              }
              frame True {
                n2746 = stacked-sequence {
                  seq-local: [w3557 _] -> [_ _]
                  seq-local: [w3556 _] -> [_ _]
                  tunnel: w3552 -> [w3559 w3589]
                  tunnel: w3551 -> [w3558 w3588]
                  tunnel: [_ w3593] -> w3550
                  tunnel: [_ w3592] -> w3549
                  frame #0 {
                    w3553 = FALSE ("布尔")
                    n2747 = local read "路径"() -> (w3555:path)
                    n2748 = Empty String/Path?(string/path=w3555) -> (empty?=w3554:bool)
                    n2749 = case shown="假" w3554 {
                      tunnel: w3559 -> [w3567 w3585]
                      tunnel: w3558 -> [w3566 w3584]
                      tunnel: [w3563 w3584] -> w3557
                      tunnel: [w3562 w3585] -> w3556
                      frame False {
                        n2750 = global read "EV05全局变量1.vi" "授权功能"() -> (w3564:bool)
                        n2751 = case shown="真" w3564 {
                          tunnel: [TRUE ("发送成功") w3576] -> w3565
                          frame False {
                          }
                          frame True {
                            n2752 = local read "设备索引号"() -> (w3570:u16)
                            n2753 = local read "CAN卡类型"() -> (w3571:u32)
                            n2754 = local read "CAN端口"() -> (w3569:u16)
                            n2755 = call "标定授权发送.vi"("CAN卡类型"=w3571, "解锁类型"=enum16{"读取", "写", "下载"}."读取", "设备索引号"=w3570, "CAN端口"=w3569, "是否连接"=TRUE, "板选择"=0, "FUNC"=u32 1) -> ("发送成功"=w3576:bool)  [unwired: 8 out]
                          }
                        }
                        n2756 = case shown="真" w3565 {
                          tunnel: w3567 -> [w3578 w3583]
                          tunnel: w3566 -> [w3577 w3582]
                          tunnel: [w3578 w3580] -> w3562
                          tunnel: [w3577 w3579] -> w3563
                          frame False {
                          }
                          frame True {
                            n2757 = Enqueue Element(queue=w3583, element="读配置文件" ("元素"), error in (no error)=w3582) -> (queue out=w3580:refnum<queue>, error out=w3579:errorcluster)  [unwired: 2 out]
                          }
                        }
                        n2758 = local write "布尔"(FALSE ("布尔")) -> ()
                        n2759 = Wait Until Next ms Multiple(millisecond multiple=u32 200 ("毫秒倍数")) -> ()  [unwired: 1 out]
                      }
                      frame True {
                      }
                    }
                    n2760 = local write "1 6"(w3553) -> ()
                    n2761 = local write "1 7"(w3553) -> ()
                    n2762 = local write "1 8"(w3553) -> ()
                    n2763 = local write "1 9"(w3553) -> ()
                    n2764 = local write "1 10"(w3553) -> ()
                    n2765 = local write "1 12"(w3553) -> ()
                  }
                  frame #1 {
                    w3586 = FALSE ("流控帧")
                    w3587 = TRUE ("流控帧 2")
                    n2766 = global read "EV05全局变量1.vi" "授权功能"() -> (w3590:bool)
                    n2767 = case shown="假" w3590 {
                      tunnel: [TRUE ("发送成功") w3602] -> w3591
                      frame False {
                      }
                      frame True {
                        n2768 = local read "设备索引号"() -> (w3596:u16)
                        n2769 = local read "CAN卡类型"() -> (w3597:u32)
                        n2770 = local read "CAN端口"() -> (w3595:u16)
                        n2771 = call "标定授权发送.vi"("CAN卡类型"=w3597, "解锁类型"=enum16{"读取", "写", "下载"}."读取", "设备索引号"=w3596, "CAN端口"=w3595, "是否连接"=TRUE, "板选择"=0, "FUNC"=u32 1) -> ("发送成功"=w3602:bool)  [unwired: 8 out]
                      }
                    }
                    n2772 = case shown="真" w3591 {
                      tunnel: w3589 -> [w3604 w3605]
                      tunnel: w3588 -> [w3603 w3608]
                      tunnel: [w3604 w3610] -> w3593
                      tunnel: [w3603 w3609] -> w3592
                      frame False {
                      }
                      frame True {
                        n2773 = Flush Queue(queue=w3605, error in (no error)=w3608) -> (queue out=w3606:refnum<queue>, error out=w3607:errorcluster)  [unwired: 1 out]
                        n2774 = Enqueue Element(queue=w3606, element="全部读取" ("元素"), error in (no error)=w3607) -> (queue out=w3610:refnum<queue>, error out=w3609:errorcluster)  [unwired: 2 out]
                      }
                    }
                    n2775 = global write "EV05全局变量1.vi" "写入超时"(w3586) -> ()
                    n2776 = global write "EV05全局变量1.vi" "流控帧"(w3586) -> ()
                    n2777 = local write "写?"(w3586) -> ()
                    n2778 = local write "消除"(w3587) -> ()
                    n2779 = local write "控制1"(w3587) -> ()
                    n2780 = global write "EV05全局变量1.vi" "流控帧 2"(w3587) -> ()
                  }
                }
              }
            }
          }
          event "开启均衡": Value Change {
            n2781 = event-data() -> ("NewVal"=w3616:bool)  [unwired: 5 out]
            n2782 = case shown="真" w3616 {
              tunnel: w3615 -> [w3618 w3625]
              tunnel: w3614 -> [w3617 w3624]
              tunnel: [w3618 w3623] -> w3613
              tunnel: [w3617 w3622] -> w3612
              frame False {
              }
              frame True {
                n2783 = global read "EV05全局变量1.vi" "授权功能"() -> (w3620:bool)
                n2784 = case shown="假" w3620 {
                  tunnel: [TRUE ("发送成功") w3635] -> w3621
                  frame False {
                  }
                  frame True {
                    n2785 = local read "主从选择"() -> (w3627:enum32{"主板", "从板"})
                    n2786 = case shown="\"从板\"" w3627 {
                      tunnel: [0.0 ("FUNC") w3637] -> w3628
                      frame "主板", Default {
                      }
                      frame "从板" {
                        n2787 = local read "从板号"() -> (w3637:u8)
                      }
                    }
                    n2788 = local read "设备索引号"() -> (w3630:u16)
                    n2789 = local read "CAN卡类型"() -> (w3631:u32)
                    n2790 = local read "CAN端口"() -> (w3629:u16)
                    n2791 = call "标定授权发送.vi"("CAN卡类型"=w3631, "解锁类型"=enum16{"读取", "写", "下载"}."写", "设备索引号"=w3630, "CAN端口"=w3629, "是否连接"=TRUE, "板选择"=0, "FUNC"=w3628) -> ("发送成功"=w3635:bool)  [unwired: 8 out]
                  }
                }
                n2792 = case shown="真" w3621 {
                  tunnel: w3625 -> [w3639 w3644]
                  tunnel: w3624 -> [w3638 w3643]
                  tunnel: [w3639 w3641] -> w3623
                  tunnel: [w3638 w3640] -> w3622
                  frame False {
                  }
                  frame True {
                    n2793 = Enqueue Element(queue=w3644, element="开启均衡" ("元素"), error in (no error)=w3643) -> (queue out=w3641:refnum<queue>, error out=w3640:errorcluster)  [unwired: 2 out]
                  }
                }
                n2794 = call <vilib>:"Set Busy.vi"("disable click? (T)"=TRUE) -> ()  [unwired: 3 in, 8 out]
              }
            }
          }
          event "关闭均衡": Value Change {
            n2795 = event-data() -> ("NewVal"=w3649:bool)  [unwired: 5 out]
            n2796 = case shown="真" w3649 {
              tunnel: w3648 -> [w3651 w3658]
              tunnel: w3647 -> [w3650 w3657]
              tunnel: [w3651 w3656] -> w3646
              tunnel: [w3650 w3655] -> w3645
              frame False {
              }
              frame True {
                n2797 = global read "EV05全局变量1.vi" "授权功能"() -> (w3653:bool)
                n2798 = case shown="假" w3653 {
                  tunnel: [TRUE ("发送成功") w3668] -> w3654
                  frame False {
                  }
                  frame True {
                    n2799 = local read "主从选择"() -> (w3660:enum32{"主板", "从板"})
                    n2800 = case shown="\"从板\"" w3660 {
                      tunnel: [0.0 ("FUNC") w3670] -> w3661
                      frame "主板", Default {
                      }
                      frame "从板" {
                        n2801 = local read "从板号"() -> (w3670:u8)
                      }
                    }
                    n2802 = local read "设备索引号"() -> (w3663:u16)
                    n2803 = local read "CAN卡类型"() -> (w3664:u32)
                    n2804 = local read "CAN端口"() -> (w3662:u16)
                    n2805 = call "标定授权发送.vi"("CAN卡类型"=w3664, "解锁类型"=enum16{"读取", "写", "下载"}."写", "设备索引号"=w3663, "CAN端口"=w3662, "是否连接"=TRUE, "板选择"=0, "FUNC"=w3661) -> ("发送成功"=w3668:bool)  [unwired: 8 out]
                  }
                }
                n2806 = case shown="真" w3654 {
                  tunnel: w3658 -> [w3672 w3677]
                  tunnel: w3657 -> [w3671 w3676]
                  tunnel: [w3672 w3674] -> w3656
                  tunnel: [w3671 w3673] -> w3655
                  frame False {
                  }
                  frame True {
                    n2807 = Enqueue Element(queue=w3677, element="关闭均衡" ("元素"), error in (no error)=w3676) -> (queue out=w3674:refnum<queue>, error out=w3673:errorcluster)  [unwired: 2 out]
                  }
                }
                n2808 = call <vilib>:"Set Busy.vi"("disable click? (T)"=TRUE) -> ()  [unwired: 3 in, 8 out]
              }
            }
          }
          event "强制开启均衡": Value Change {
            n2809 = event-data() -> ("NewVal"=w3682:bool)  [unwired: 5 out]
            n2810 = case shown="真" w3682 {
              tunnel: w3681 -> [w3684 w3691]
              tunnel: w3680 -> [w3683 w3690]
              tunnel: [w3684 w3689] -> w3679
              tunnel: [w3683 w3688] -> w3678
              frame False {
              }
              frame True {
                n2811 = global read "EV05全局变量1.vi" "授权功能"() -> (w3686:bool)
                n2812 = case shown="假" w3686 {
                  tunnel: [TRUE ("发送成功") w3701] -> w3687
                  frame False {
                  }
                  frame True {
                    n2813 = local read "主从选择"() -> (w3693:enum32{"主板", "从板"})
                    n2814 = case shown="\"从板\"" w3693 {
                      tunnel: [0.0 ("FUNC") w3703] -> w3694
                      frame "主板", Default {
                      }
                      frame "从板" {
                        n2815 = local read "从板号"() -> (w3703:u8)
                      }
                    }
                    n2816 = local read "设备索引号"() -> (w3696:u16)
                    n2817 = local read "CAN卡类型"() -> (w3697:u32)
                    n2818 = local read "CAN端口"() -> (w3695:u16)
                    n2819 = call "标定授权发送.vi"("CAN卡类型"=w3697, "解锁类型"=enum16{"读取", "写", "下载"}."写", "设备索引号"=w3696, "CAN端口"=w3695, "是否连接"=TRUE, "板选择"=0, "FUNC"=w3694) -> ("发送成功"=w3701:bool)  [unwired: 8 out]
                  }
                }
                n2820 = case shown="真" w3687 {
                  tunnel: w3691 -> [w3705 w3710]
                  tunnel: w3690 -> [w3704 w3709]
                  tunnel: [w3705 w3707] -> w3689
                  tunnel: [w3704 w3706] -> w3688
                  frame False {
                  }
                  frame True {
                    n2821 = Enqueue Element(queue=w3710, element="强制均衡" ("元素"), error in (no error)=w3709) -> (queue out=w3707:refnum<queue>, error out=w3706:errorcluster)  [unwired: 2 out]
                  }
                }
                n2822 = call <vilib>:"Set Busy.vi"("disable click? (T)"=TRUE) -> ()  [unwired: 3 in, 8 out]
              }
            }
          }
        }
        n2823 = Unbundle By Name(w922) -> ("status"=w921:bool)
        n2824 = Or(x=w921, y=w923) -> (x .or. y?=w924:bool)
      }
      n2825 = Release Queue(queue=w917, force destroy? (F)=TRUE ("强制销毁？(F)"), error in (no error)=w916) -> (error out=w914:errorcluster)  [unwired: 2 out]
      n2826 = call <vilib>:"Clear Errors.vi"("error in (no error)"=w914) -> ()  [unwired: 7 out]
    }
    frame Disabled {
    }
  }
  n2827 = while {
    tunnel: w60 -> [w3722]
